vi "Read Graph Data.vi"(11 "Harmonics in":refnum<class "Harmonics.lvclass">) -> (2 "Graph Data":cluster{"Array":dbl[], "Array":dbl[]}[](array[cluster]), 3 "Harmonics out":refnum<class "Harmonics.lvclass">)   [LabVIEW 2020, in "Harmonics.lvclass"]
uses:
  Harmonics.lvclass
  Harmonics.lvclass/Harmonics.ctl
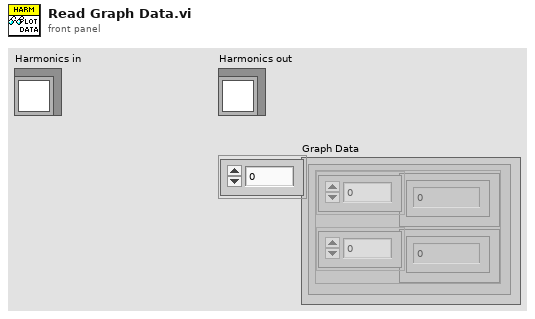
[diagram p1: front panel]
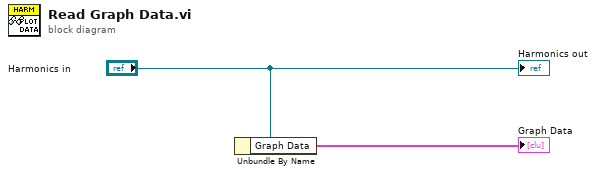
[diagram p0: block diagram]
diagram:
  n1 = Unbundle By Name("Harmonics in") -> ("Graph Data"=→"Graph Data":cluster{"Array":dbl[], "Array":dbl[]}[])
  "Harmonics out" <- "Harmonics in"
